vi "test_slide-fill-color.vi"() -> ()   [LabVIEW 2019]
panel:
  in  "limit":dbl(slide) scale=0.0..10.0
  in  "stop":bool
  in  "input":dbl(slide) scale=0.0..10.0
  out "Slide":dbl(slide) scale=0.0..10.0
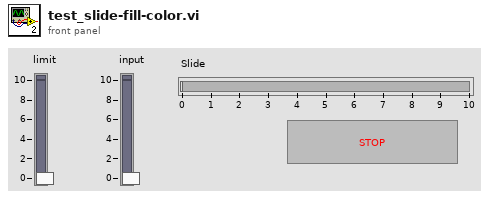
[diagram p1: front panel]
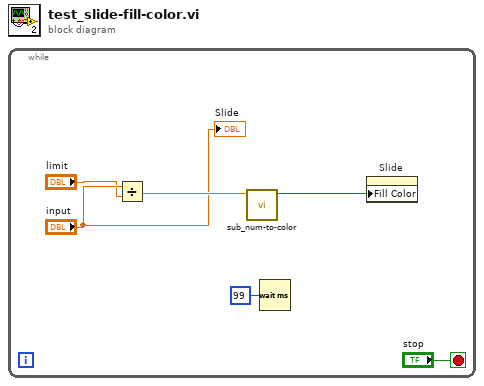
[diagram p0: block diagram]
diagram:
  n1 = while {
    stop <- "stop" stop-if-true
    n2 = Divide(x="input", y="limit") -> (x/y=w3:dbl)
    n3 = call "sub_num-to-color.vi"("ratio"=w3) -> ("color num"=w6:u32)  [unwired: 10 in]
    n4 = Wait (ms)(milliseconds to wait=u32 99) -> ()  [unwired: 1 out]
    n5 = property on="Slide" class="Slide (strict)"("Fill Color"=w6) -> ()  [unwired: 2 in, 2 out]
    "Slide" <- "input"
  }
